vi "Init Actor Core.vi"(8 "error in (no error)":errorcluster, 11 "Measure Object in":refnum<class "Spectrum Recorder too.lvclass">) -> (0 "error out":errorcluster, 3 "Measure Object out":refnum<class "Spectrum Recorder too.lvclass">)   [LabVIEW 2016, in "Spectrum Recorder too.lvclass"]
uses:
  Spectrum Recorder too.lvclass
  C:/github/LabActor/Worker/Worker.lvclass
  Worker/Worker.lvclass/Worker.ctl
  Worker/Write File prefix.vi
  Instrument Actor/Instrument Actor.lvclass
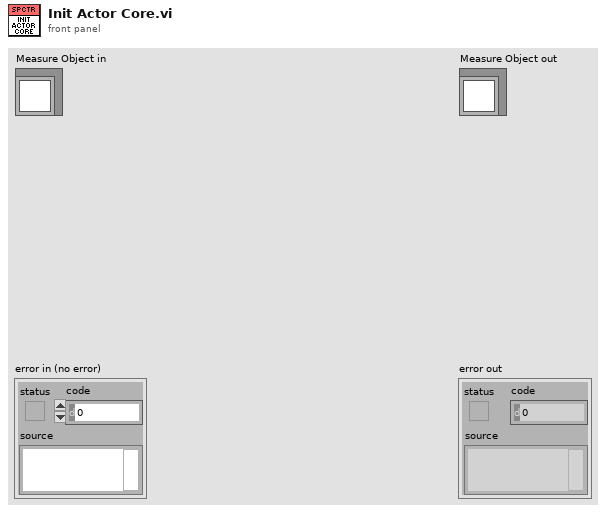
[diagram p1: front panel]
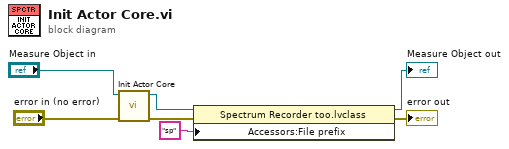
[diagram p0: block diagram]
diagram:
  n1 = call-parent "Init Actor Core.vi"("error in (no error)"="error in (no error)", "Measure Object in"="Measure Object in") -> ("error out"=w7:errorcluster, "Measure Object out"=w3:refnum<class "Spectrum Recorder too.lvclass">)  [unwired: 8 in]
  n2 = property class="Spectrum Recorder too.lvclass"(reference=w3, error in=w7, "Accessors:File prefix"="sp" ("File prefix")) -> (reference out=→"Measure Object out":refnum<class "Spectrum Recorder too.lvclass">, error out=→"error out":errorcluster)
